vi "~Read Four positions with two reads.vi"   [LabVIEW 2017]
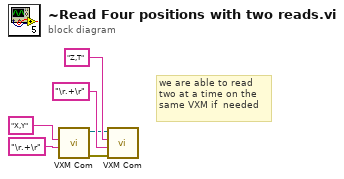
[diagram p0: block diagram]
diagram:
  # "we are able to read \ntwo at a time on the\nsame VXM if  needed"
  n1 = call "VXM Com.vi"("Termination String ('/' codes)"="\r.+\r", "Write Buffer ('/' codes)"="X,Y" ("Write Buffer")) -> ("error out"=w1:errorcluster, "VISA resource out"=w2:refnum<visa-resource-name>)  [unwired: 7 in, 1 out]
  n2 = call "VXM Com.vi"("error in (no error)"=w1, "Termination String ('/' codes)"="\r.+\r", "Write Buffer ('/' codes)"="Z,T" ("Write Buffer"), "VISA resource name"=w2) -> ()  [unwired: 5 in, 3 out]
